vi "MM6.InitCleanAfg.vi"(0 "i ref in":refnum<vi>, 2 "InitObjs":string[](array[string]), 3 "ms timeout (10000)":i32=10000, 5 "error in (no error)":errorcluster) -> (14 "i ref out":refnum<vi>, 16 "InitObjs out":string[](array[string]), 17 "timed out":bool, 19 "error out":errorcluster)   [LabVIEW 2014, in "MM6.lvlib"]
doc: "Initializes the \"CleanHandler\"."
uses:
  MM6.lvlib
  CSCore/CSSystem/CoreLib/CoreLib.double 2 byte array.vi
  CSCore/CSSystem/CoreLib/CoreLib.int 2 byte array.vi
  CSCore/BaseProcess/BaseProcess.lvlib
  LEBITLib/LEBITLib.lvlib
  CSCore/CSSystem/CoreLib/CoreLib.lvlib
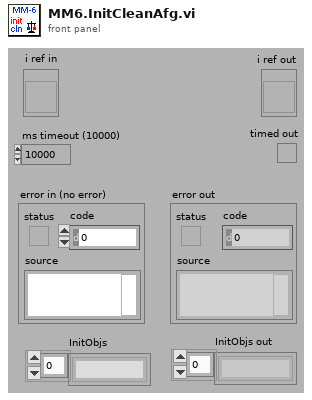
[diagram p1: front panel]
types:
  T1 = enum16{"simple", "synchronous", "asynchronous", "notification"}
  T2 = typedef "MM6.lvlib/MM6.i attribute.ctl" = cluster{"ConfigData":T3, "UsedObjs":string[], "ActScanStep":i32[], "AbortRequest":bool, "StopRequest":bool, "# cycles":i32, "Connected":bool, "MMStatus":T18, "# data":i32, "DIMServices":cluster{"MM6StatusString":string, "MM6StatusID":i32, "discArchiver":string, "discArchiverID":i32, "eventBuilder":string, "eventBuilderID":i32, "GUIIDString":string, "GUIIDStringID":i32}, "dataFile":string, "ExtraDataSets":T19, "PGRunning":T20}
  T3 = typedef "LEBITDefs.lvlib/LEBITDefs.ConfigData.ctl" = cluster{"GenConfig":T4, "Configs":T6[]}
  T4 = typedef "LEBITDefs.lvlib/LEBITDefs.GenConfig.ctl" = cluster{"Mode":i32, "Logs":T5[]}
  T5 = typedef "LEBITDefs.lvlib/LEBITDefs.Log.ctl" = cluster{"Name":string, "FctName":string, "Special":string}
  T6 = typedef "LEBITDefs.lvlib/LEBITDefs.OneConfig.ctl" = cluster{"MCA":T7, "Timing":T8, "Scans":T11[], "FreqDevs":T12[], "CleanDev":T13, "NrCycles":i32, "Specials":T15[], "Delays":T16[], "DAC":T17}
  T7 = typedef "LEBITDefs.lvlib/LEBITDefs.MCA.ctl" = cluster{"Name":string, "Address":string, "NrChannels":i32, "Gate":i32, "NrPipse":i32}
  T8 = typedef "LEBITDefs.lvlib/LEBITDefs.Timing.ctl" = cluster{"TimeTables":cluster{"TimeTable":T9}[], "Memories":T10[], "ScanX":string, "ScanY":string}
  T9 = typedef "LEBITDefs.lvlib/LEBITDefs.Timetable.ctl" = dbl[]
  T10 = typedef "LEBITDefs.lvlib/LEBITDefs.Memory.ctl" = cluster{"Device":string, "ExtTrig":bool, "TT2Use":i32, "PatternTable":string[]}
  T11 = typedef "LEBITDefs.lvlib/LEBITDefs.ScanDev.ctl" = cluster{"Name":string, "FctName":string, "Values":dbl[], "NrScanVals":i32, "Special":string}
  T12 = typedef "LEBITDefs.lvlib/LEBITDefs.FreqDev.ctl" = cluster{"Name":string, "Amp":dbl, "CenterFreq":dbl, "Time":dbl}
  T13 = typedef "LEBITDefs.lvlib/LEBITDefs.CleanDev.ctl" = cluster{"Name":string, "CleanData":T14[]}
  T14 = typedef "LEBITDefs.lvlib/LEBITDefs.CleanDataType.ctl" = cluster{"Amp":dbl, "Center":dbl, "Plus":dbl, "Minus":dbl, "Time":dbl}
  T15 = typedef "LEBITDefs.lvlib/LEBITDefs.Special.ctl" = cluster{"Name":string, "FctName":string, "VerySpecial":string, "Data":dbl}
  T16 = typedef "LEBITDefs.lvlib/LEBITDefs.Delay.ctl" = cluster{"Name":string, "Delay":dbl}
  T17 = typedef "LEBITDefs.lvlib/LEBITDefs.DAC.ctl" = cluster{"Name":string, "Step1":i32, "Step2":i32}
  T18 = typedef "MM6.lvlib/MM6.status.ctl" = enum16{"loaded", "load_error", "config", "config_error", "init", "init_error", "data_reset", "data_reset_error", "running", "start_error", "run_error", "abort_requested", "aborted", "stop_requested", "stopped", "stop_error", "Connected", "NOTConnected"}
  T19 = typedef "LEBITDefs.lvlib/LEBITDefs.ExtraData.ctl" = cluster{"Ions":cluster{"ExcitIonMass":string, "ExcitIonCharge":i32, "CleanIons":cluster{"CleanIonMass":string, "CleanIonCharge":i32}[]}, "TimingDescription":cluster{"TimeTableDescription":cluster{"Times":string[]}[], "PatternTableDescription":cluster{"Pattern":string[]}[]}, "ScanUnits":string[]}[]
  T20 = typedef "PPG_ABC.lvlib/PPG_ABC.PG_Running.ctl" = i32
  T21 = typedef "CoreDefs.rawDataType.ctl" = i8[]
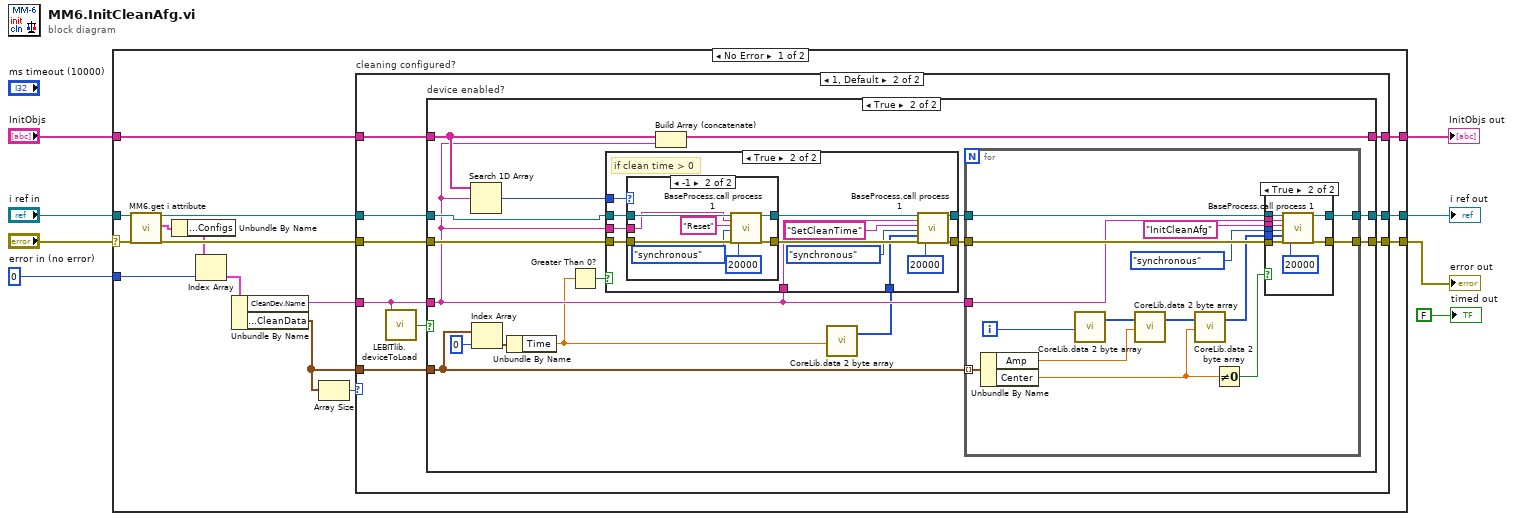
[diagram p0: block diagram]
diagram:
  n1 = case shown="No Error" "error in (no error)" {
    selector: "error in (no error)" -> [w15 w106]
    tunnel: "i ref in" -> [w20 w107]
    tunnel: [w19 w107] -> w7
    tunnel: [w18 w106] -> w6
    tunnel: "InitObjs" -> [w17 w108]
    tunnel: [w16 w108] -> w3
    tunnel: 0 ("index") -> [w10 _]
    frame No Error {
      n2 = call "MM6.get i attribute.vi"("i ref in"=w20, "error in (no error)"=w15) -> ("i ref out"=w22:refnum<vi>, "i attribute"=w12:T2, "error out"=w21:errorcluster)  [unwired: 15 in]
      n3 = Unbundle By Name(w12) -> ("ConfigData.Configs"=w11:T6[])
      n4 = Index Array(array=w11, index=w10) -> (element=w9:T6)
      n5 = Unbundle By Name(w9) -> ("CleanDev.Name"=w14:string, "CleanDev.CleanData"=w13:T14[])
      n6 = Array Size(array=w13) -> (size(s)=w23:i32)
      n7 = case "cleaning configured?" shown="1, Default" w23 {
        tunnel: w22 -> [w26 w35]
        tunnel: [w26 w34] -> w19
        tunnel: w21 -> [w25 w33]
        tunnel: [w25 w32] -> w18
        tunnel: w17 -> [w24 w31]
        tunnel: [w24 w30] -> w16
        tunnel: w14 -> [_ w27]
        tunnel: w13 -> [_ w29]
        frame 0 {
        }
        frame 1, Default {
          n8 = call "LEBITlib.deviceToLoad.vi"("DeviceName"=w27) -> ("DeviceIsToLoad"=w28:bool)
          n9 = case "device enabled?" shown="True" w28 {
            tunnel: w35 -> [w38 w54]
            tunnel: [w38 w45] -> w34
            tunnel: w33 -> [w37 w53]
            tunnel: w27 -> [_ w42]
            tunnel: [w37 w44] -> w32
            tunnel: w31 -> [w36 w51]
            tunnel: [w36 w50] -> w30
            tunnel: w29 -> [_ w47]
            frame False {
            }
            frame True {
              n10 = Search 1D Array(1D array=w51, element=w42) -> (index of element=w52:i32)  [unwired: 1 in]
              n11 = Index Array(array=w47, index=0) -> (element=w49:T14)
              n12 = Unbundle By Name(w49) -> ("Time"=w39:dbl)
              n13 = Greater Than 0?(x=w39) -> (x > 0?=w41:bool)
              n14 = Build Array (concatenate)(w51, w42) -> (w50:string[])
              n15 = call-poly "CoreLib.data 2 byte array.vi"("f64"=w39) -> ("byteArray out"=w40:T21)  [unwired: 18 in]
              n16 = case shown="True" w41 {
                tunnel: w54 -> [w56 w69]
                tunnel: w53 -> [w55 w68]
                tunnel: w52 -> [_ w65]
                tunnel: [w56 w62] -> w46
                tunnel: [w55 w61] -> w43
                tunnel: w42 -> [_ w60]
                tunnel: w42 -> [_ w58]
                tunnel: w40 -> [_ w57]
                frame False {
                  # "clean time = 0 -> no cleaning"
                }
                frame True {
                  # "if clean time > 0"
                  n17 = case shown="-1" w65 {
                    tunnel: w69 -> [w71 w79]
                    tunnel: w68 -> [w70 w78]
                    tunnel: [w71 w77] -> w67
                    tunnel: [w70 w76] -> w66
                    tunnel: w60 -> [_ w74]
                    frame 0, Default {
                    }
                    frame -1 {
                      n18 = call "BaseProcess.call process 1.vi"("i ref in"=w79, "Object"=w74, "Selector"="Reset", "CallType"=T1."synchronous", "error in (no error)"=w78, "timeout (ms)"=20000) -> ("i ref out"=w77:refnum<vi>, "error out"=w76:errorcluster)  [unwired: 11 in, 1 out]
                    }
                  }
                  n19 = call "BaseProcess.call process 1.vi"("i ref in"=w67, "Object"=w58, "Selector"="SetCleanTime", "CallType"=T1."synchronous", "Data"=w57, "error in (no error)"=w66, "timeout (ms)"=20000) -> ("i ref out"=w62:refnum<vi>, "error out"=w61:errorcluster)  [unwired: 10 in, 1 out]
                }
              }
              n20 = for {
                tunnel: w47 -> [w89] mode=indexing
                tunnel: w46 -> [w94]
                tunnel: [w93] -> w45
                tunnel: [w92] -> w44
                tunnel: w43 -> [w91]
                tunnel: w42 -> [w90]
                i -> [w81]
                n21 = Unbundle By Name(w89) -> ("Amp"=w80:dbl, "Center"=w82:dbl)
                n22 = call-poly "CoreLib.data 2 byte array.vi"("i32"=w81) -> ("byteArray out"=w85:T21)  [unwired: 18 in]
                n23 = call-poly "CoreLib.data 2 byte array.vi"("byteArray"=w85, "f64"=w80) -> ("byteArray out"=w83:T21)  [unwired: 17 in]
                n24 = call-poly "CoreLib.data 2 byte array.vi"("byteArray"=w83, "f64"=w82) -> ("byteArray out"=w84:T21)  [unwired: 17 in]
                n25 = Not Equal To 0?(x=w82) -> (x != 0?=w86:bool)
                n26 = case shown="True" w86 {
                  tunnel: w94 -> [w96 w104]
                  tunnel: [w96 w103] -> w93
                  tunnel: [w95 w102] -> w92
                  tunnel: w91 -> [w95 w101]
                  tunnel: w90 -> [_ w100]
                  tunnel: "InitCleanAfg" ("Selector") -> [_ w99]
                  tunnel: T1."synchronous" ("CallType") -> [_ w98]
                  tunnel: w84 -> [_ w97]
                  frame False {
                  }
                  frame True {
                    n27 = call "BaseProcess.call process 1.vi"("i ref in"=w104, "Object"=w100, "Selector"=w99, "CallType"=w98, "Data"=w97, "error in (no error)"=w101, "timeout (ms)"=20000) -> ("i ref out"=w103:refnum<vi>, "error out"=w102:errorcluster)  [unwired: 10 in, 1 out]
                  }
                }
              }
            }
          }
        }
      }
    }
    frame Error {
    }
  }
  "error out" <- w6
  "i ref out" <- w7
  "InitObjs out" <- w3
  "timed out" <- FALSE ("timed out")
